vi "CoordRunAnalysis.vi"(0 "Refnum in":T3, 1 "CoordinatteEntry In":T4 {"CaliperSetting"."CaliperEntry"."CaliperType" items=["Distance", "Mid Point", "Perpendicular Projection", "Lines Intersection", "Angle from Horizontal", "Angle from Vertical", "Angle Defined by 3 Points", "Angle Defined by 4 Points", "Bissecting Line", "Mid Line", "Center of Mass", "Area", "Line Fit", "Circle Fit", "Ellipse Fit"]; "OriginPointInfo"."Mode" items=["Horizontal Motion", "Vertical Motion", "Horizontal and Vertical Motion", "Horizontal. Vertical and Angular Motion"]; "AnalysisSetting"."ROI"."Contours"."Type" items=["No Selection", "Point", "Line", "Rectangle", "Oval", "Polygon", "Freehand Region", "Annulus", "Unused2", "Unused3", "Broken Line", "Freehand Line", "Rotated Rectangle"]}, 4 "AnalysisSetting":T1[](array[typedef]) {"ROI"."Contours"."Type" items=["No Selection", "Point", "Line", "Rectangle", "Oval", "Polygon", "Freehand Region", "Annulus", "Unused2", "Unused3", "Broken Line", "Freehand Line", "Rotated Rectangle"]}, 5 "Error In":errorcluster, 7 "CoordSystemRun?":bool, 9 "CreatDllImage":bool, 11 "RootPath":path, 13 "Dllindex":i32) -> (12 "AnalysisCoor":bool, 15 "CoordinatteEntry Out":T4 {"CaliperSetting"."CaliperEntry"."CaliperType" items=["Distance", "Mid Point", "Perpendicular Projection", "Lines Intersection", "Angle from Horizontal", "Angle from Vertical", "Angle Defined by 3 Points", "Angle Defined by 4 Points", "Bissecting Line", "Mid Line", "Center of Mass", "Area", "Line Fit", "Circle Fit", "Ellipse Fit"]; "OriginPointInfo"."Mode" items=["Horizontal Motion", "Vertical Motion", "Horizontal and Vertical Motion", "Horizontal. Vertical and Angular Motion"]; "AnalysisSetting"."ROI"."Contours"."Type" items=["No Selection", "Point", "Line", "Rectangle", "Oval", "Polygon", "Freehand Region", "Annulus", "Unused2", "Unused3", "Broken Line", "Freehand Line", "Rotated Rectangle"]}, 18 "Main Out":T13[](array[typedef]), 19 "Error Out":errorcluster)   [LabVIEW 2019]
uses:
  Analysis/Controls/Analysis_Setting.ctl
  Process/Controls/Process_Setting.ctl
  Controls/Vision_DataEntry.ctl
  Control/DataTransform.ctl
  Analysis/Controls/Analysis_Result_To_Caliper.ctl
  Caliper/Controls/AnalysisResultPointsAction.ctl
  Analysis/Controls/V_Analysis_Type.ctl
  Ctrl/VisionProcessName.ctl
  Control/CoordinateAnalysisSetting.ctl
  Control/CoordinatteEntry.ctl
  <vilib>/vision/Image Controls.llb/IMAQ Image.ctl
  Caliper/Controls/CaliperType.ctl
  Caliper/Controls/SelectionListEntryPointType.ctl
  Caliper/Controls/SelectionListEntry.ctl
  Control/CoordinateCaliperSetting.ctl
  Caliper/Controls/CaliperResult.ctl
  Caliper/Controls/CaliperDataEntry.ctl
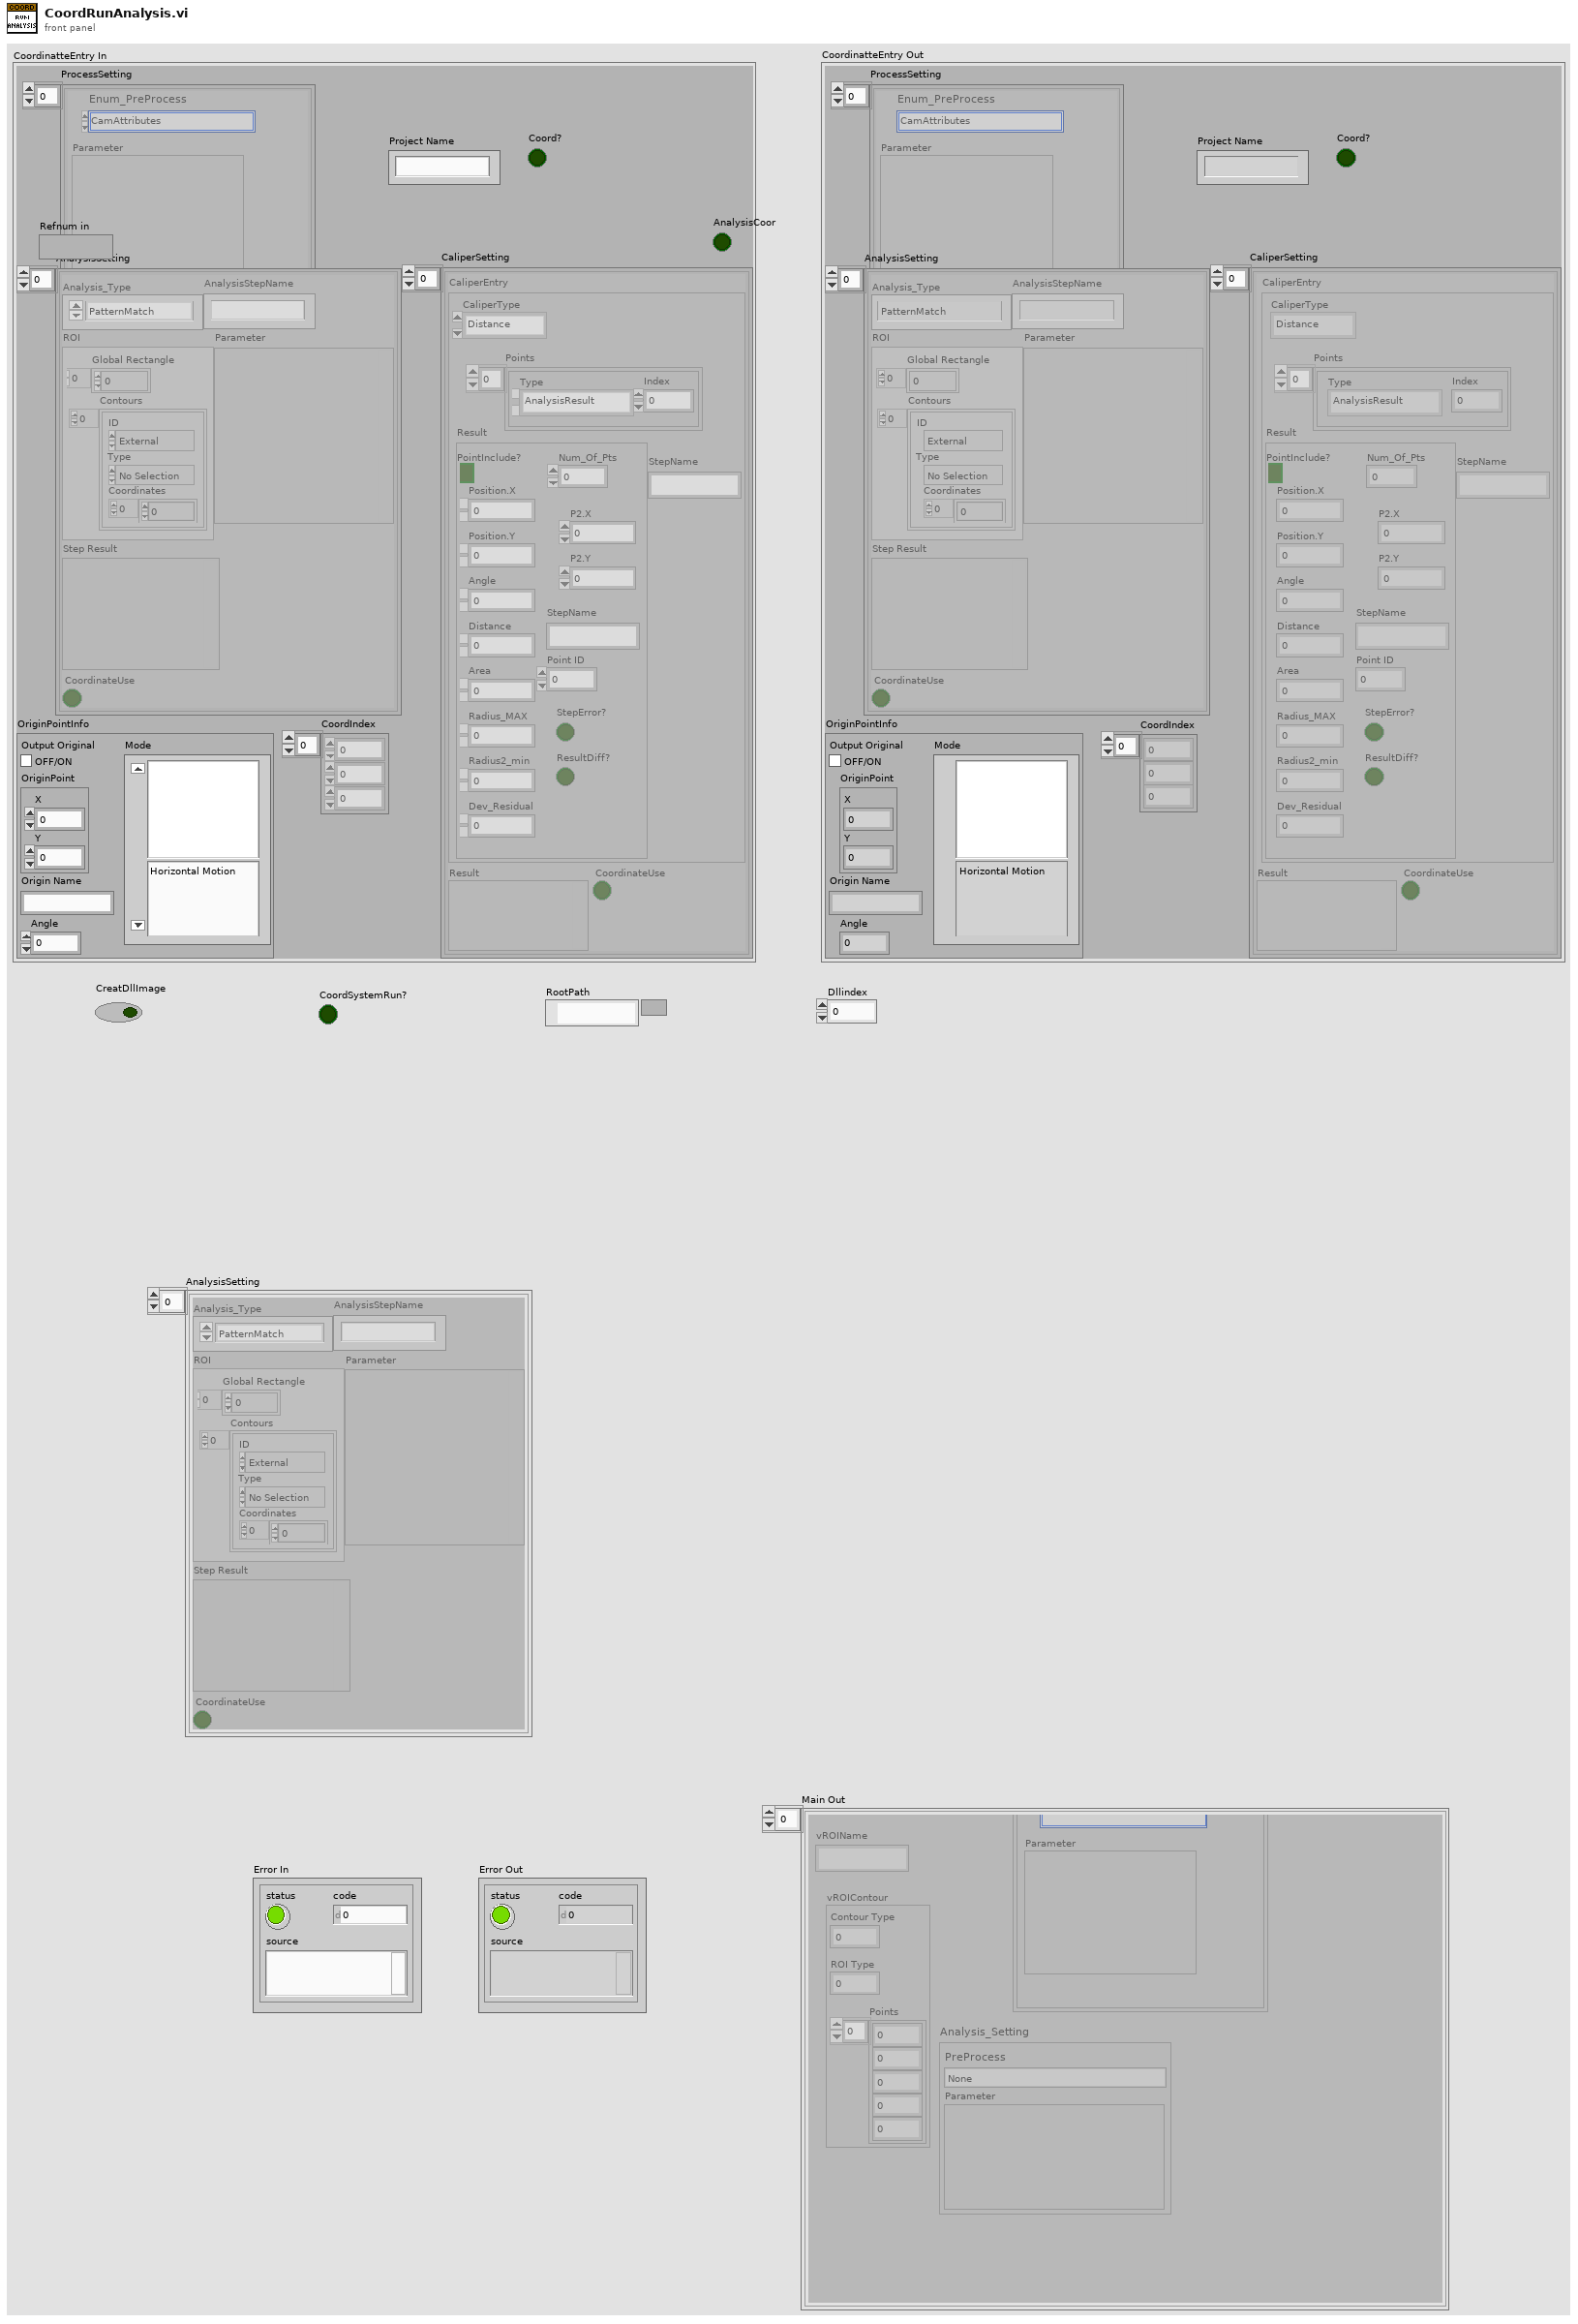
[diagram p1: front panel]
types:
  T1 = typedef "CoordinateAnalysisSetting.ctl" = cluster{"Analysis_Type":enum16{"PatternMatch", "Straight Edge"}, "ROI ":T2, "Parameter":variant, "Step Result":variant, "AnalysisStepName":string, "CoordinateUse":bool}
  T2 = typedef "ROI Descriptor" = cluster{"Global Rectangle":i32[], "Contours":cluster{"ID":enum32{"External", "Internal"}, "Type":u32, "Coordinates":i32[]}[]}
  T3 = typedef "IMAQ Image.ctl" = refnum<image>
  T4 = typedef "CoordinatteEntry.ctl" = cluster{"ProcessSetting":T5[], "Project Name":string, "AnalysisSetting":T1[], "Coord?":bool, "OriginPointInfo":cluster{"Output Original":bool, "Origin Name":string, "Angle":dbl, "Mode":u16, "OriginPoint":cluster{"X":dbl, "Y":dbl}}, "CaliperSetting":T7[], "CoordIndex":i32[]}
  T5 = typedef "Process_Setting.ctl" = cluster{"Enum_PreProcess":T6, "Parameter":string}
  T6 = typedef "VisionProcessName.ctl" = enum16{"*CamParameter*", "CamAttributes", "*Preprocess*", "CG_Brightness", "C_Plane Extraction", "C_Threshold", "G_Lookup Table", "G_Threshold"}
  T7 = typedef "CoordinateCaliperSetting.ctl" = cluster{"Result":variant, "CoordinateUse":bool, "CaliperEntry":T8}
  T8 = typedef "CaliperDataEntry.ctl" = cluster{"CaliperType":T9, "Points":T10[], "Result":T12, "StepName":string}
  T9 = typedef "CaliperType.ctl" = u32
  T10 = typedef "SelectionListEntry.ctl" = cluster{"Type":T11, "Index":i32}
  T11 = typedef "SelectionListEntryPointType.ctl" = enum16{"AnalysisResult", "CaliperResult"}
  T12 = typedef "CaliperResult.ctl" = cluster{"PointInclude?":bool, "Num_Of_Pts":u8, "Position.X":dbl, "Position.Y":dbl, "Angle":dbl, "Distance":dbl, "Area":dbl, "Radius_MAX":dbl, "Radius2_min":dbl, "Dev_Residual":dbl, "P2.X":dbl, "P2.Y":dbl, "StepName":string, "Point ID":u8, "StepError?":bool, "ResultDiff?":bool}
  T13 = typedef "Vision_DataEntry.ctl" = cluster{"vROIName":string, "vROIContour":cluster{"Contour Type":u32, "ROI Type":u32, "Points":i32[]}, "ProcessSetting":T5[], "Analysis_Setting":T14}
  T14 = typedef "Analysis_Setting.ctl" = cluster{"PreProcess":T15, "Parameter":string}
  T15 = typedef "V_Analysis_Type.ctl" = enum16{"None", "C_Color Pattern Matching", "G_PatternMatching", "G_ShapeDectect", "G_GeometricMatch", "B_Area Check"}
  T16 = typedef "AnalysisResultPointsAction.ctl" = enum16{"Init", "Add", "Delete", "ReplaceAll", "ReadAll", "Close"}
  T17 = typedef "Analysis_Result_To_Caliper.ctl" = cluster{"PointName":string, "Position_X":dbl, "Position_Y":dbl}
  T18 = typedef "DataTransform.ctl" = enum16{"CoordToMain", "MainToCoord"}
  T19 = cluster{"Point1 (Pixels)":cluster{"X":sgl, "Y":sgl}, "Point2 (Pixels)":cluster{"X":sgl, "Y":sgl}, "Point1 (Real-World)":cluster{"X":sgl, "Y":sgl}, "Point2 (Real-World)":cluster{"X":sgl, "Y":sgl}, "Angle (Pixel)":dbl, "Angle (Real-World)":dbl, "Score":dbl, "Straightness":dbl, "Average SNR (db)":dbl, "Calibration Valid":bool}[]
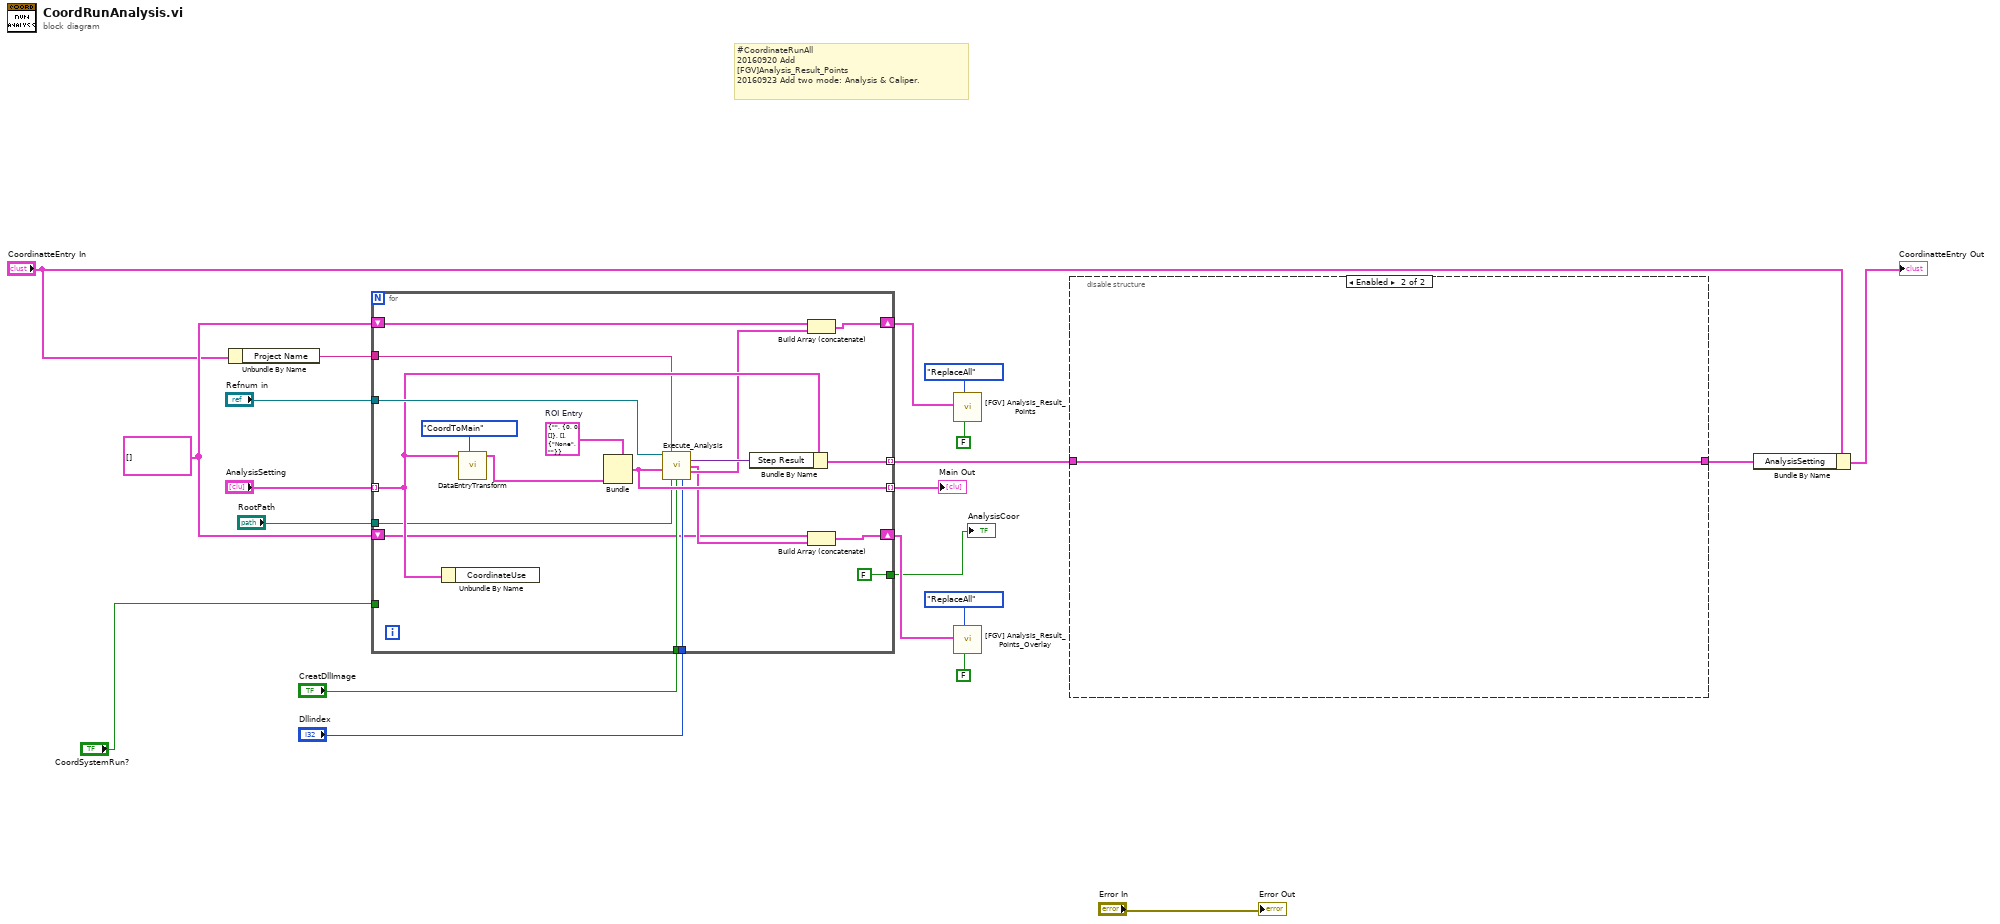
[diagram p0: block diagram]
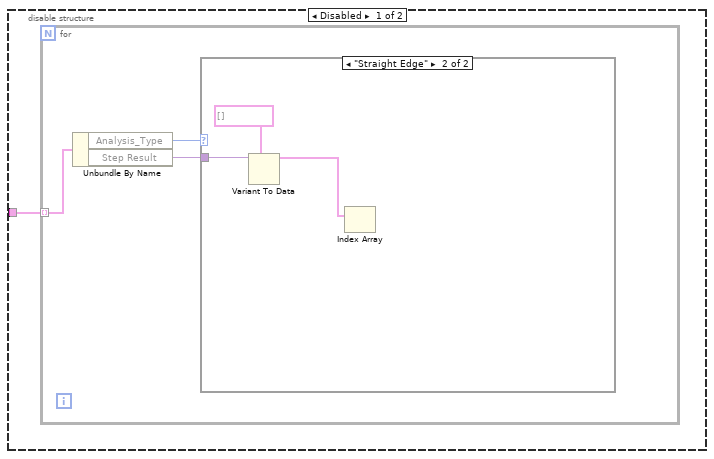
[diagram p2: hidden frame]
diagram:
  w12 = T17[] [] ("Analysis_Point_Result Out Overlay")
  # "#CoordinateRunAll\n20160920 Add\n[FGV]Analysis_Result_Points\n20160923 Add two mode: Analysis & Caliper."
  n1 = Unbundle By Name("CoordinatteEntry In") -> ("Project Name"=w18:string)
  n2 = for {
    tunnel: "AnalysisSetting" -> [w33] mode=indexing
    tunnel: "Refnum in" -> [w37]
    tunnel: [w36] -> w2 mode=indexing
    tunnel: [w34] -> w21 mode=indexing
    tunnel: "CoordSystemRun?" -> [_]
    tunnel: w18 -> [w32]
    tunnel: "RootPath" -> [w31]
    tunnel: "CreatDllImage" -> [w30]
    tunnel: "Dllindex" -> [w29]
    shift-right: [w27] -> w6
    shift-left: w12 -> [w28]
    shift-right: [w23] -> w11
    shift-left: w12 -> [w24]
    tunnel: [FALSE ("CoordinateUse")] -> w5
    w40 = T13 {"vROIName"="", "vROIContour"={"Contour Type"=0, "ROI Type"=0, "Points"=[]}, "ProcessSetting"=[], "Analysis_Setting"={"PreProcess"=enum."None", "Parameter"=""}}  # ROI Entry
    n3 = Unbundle By Name(w33) -> ()  [unwired: 1 out]
    n4 = call "DataEntryTransform.vi"("DataTrasform"=DataTransform."CoordToMain", "CoordSettingIn"=w33) -> ("MainSettingOut"=w38:T14)  [unwired: 7 in, 2 out]
    n5 = Bundle(cluster=w40, "Analysis_Setting"=w38) -> (w34:T13)  [unwired: 3 in]
    n6 = call "Execute_Analysis.vi"("Image In"=w37, "ProjectName"=w32, "ROI Entry"=w34, "RootPath"=w31, "CreatDllImage"=w30, "Script Index"=w29) -> ("Result"=w35:variant, "Analysis_Point_Result Out Overlay"=w25:T17[], "Analysis_Point_Result Out"=w26:T17[])  [unwired: 5 in, 2 out]
    n7 = Bundle By Name(cluster=w33, "Step Result"=w35) -> (w36:T1)
    n8 = Build Array (concatenate)(w28, w26) -> (w27:T17[])
    n9 = Build Array (concatenate)(w24, w25) -> (w23:T17[])
  }
  "Main Out" <- w21
  "AnalysisCoor" <- w5
  n10 = call "[FGV] Analysis_Result_Points.vi"("CoordSystemRun"=FALSE, "Action"=AnalysisResultPointsAction."ReplaceAll", "Analysis_Point_Result"=w6) -> ()  [unwired: 7 in, 2 out]
  n11 = call "[FGV] Analysis_Result_Points_Overlay.vi"("CoordSystemRun"=FALSE, "Action"=AnalysisResultPointsAction."ReplaceAll", "Analysis_Point_Result"=w11) -> ()  [unwired: 7 in, 2 out]
  n12 = disable-structure shown="Enabled" {
    disable-tunnel: w2 -> [w41 w48]
    disable-tunnel: [_ w48] -> w1
    frame Disabled {
      n13 = for {
        tunnel: w41 -> [w44] mode=indexing
        n14 = Unbundle By Name(w44) -> ("Analysis_Type"=w43:enum16{"PatternMatch", "Straight Edge"}, "Step Result"=w42:variant)
        n15 = case shown="\"Straight Edge\"" w43 {
          tunnel: w42 -> [_ w47]
          frame "PatternMatch", Default {
          }
          frame "Straight Edge" {
            n16 = Variant To Data(type=T19 [] ("Straight Edge Cluster Array"), Variant=w47) -> (data=w45:T19)  [unwired: 1 in, 1 out]
            n17 = Index Array(array=w45) -> ()  [unwired: 1 in, 1 out]
          }
        }
      }
    }
    frame Enabled {
    }
  }
  n18 = Bundle By Name(cluster="CoordinatteEntry In", "AnalysisSetting"=w1) -> (→"CoordinatteEntry Out":T4)
  "Error Out" <- "Error In"
